vi "ViewDatabase.vi"(8 "error in (no error)":errorcluster, 11 "Person in":refnum<class "Person.lvclass">) -> (0 "error out":errorcluster, 3 "Person out":refnum<class "Person.lvclass">)   [LabVIEW 2014, in "Person.lvclass"]
uses:
  Person.lvclass
  Person.lvclass/Person.ctl
  PermissionState_Interface/PermissionState.lvclass
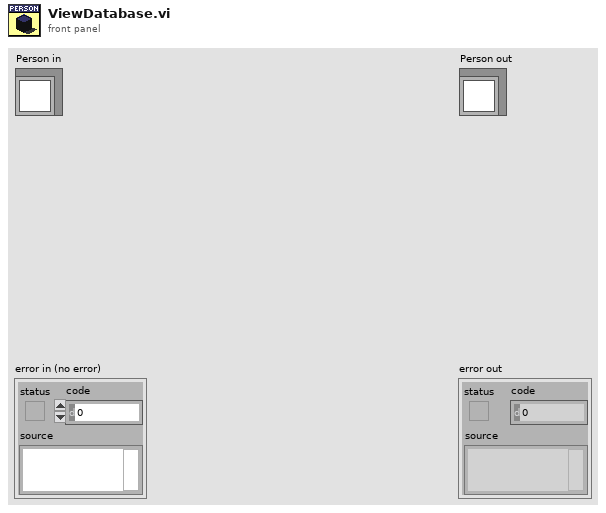
[diagram p1: front panel]
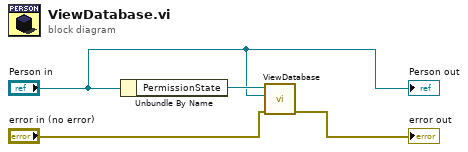
[diagram p0: block diagram]
diagram:
  n1 = Unbundle By Name("Person in") -> ("PermissionState"=w4:refnum<class "PermissionState.lvclass">)
  n2 = call-dynamic "ViewDatabase.vi"("error in (no error)"="error in (no error)", "Person in"="Person in", "PermissionState in"=w4) -> ("error out"=→"error out":errorcluster)  [unwired: 6 in, 2 out]
  "Person out" <- "Person in"
